vi "lookup_edge.vi"(9 "destination":refnum<class "Node.lvclass">, 10 "source":refnum<class "Node.lvclass">, 11 "digraph in":refnum<class "Graph.lvclass">) -> (1 "edge":refnum<class "Edge.lvclass">, 2 "edge not found?":bool)   [LabVIEW 2020, in "graph.lvlib" / "Graph.lvclass"]
uses:
  Graph.lvclass
  Node/Node.lvclass
  Edge/Edge.lvclass
  Node/Node.lvclass/Node.ctl
  Graph.lvclass/Graph.ctl
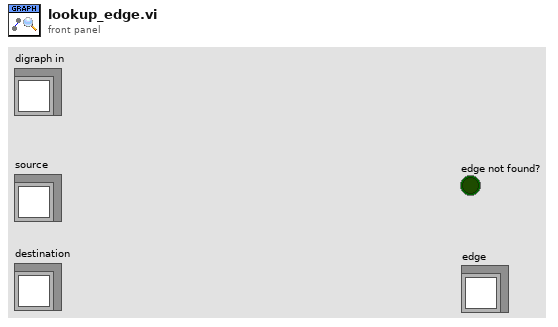
[diagram p1: front panel]
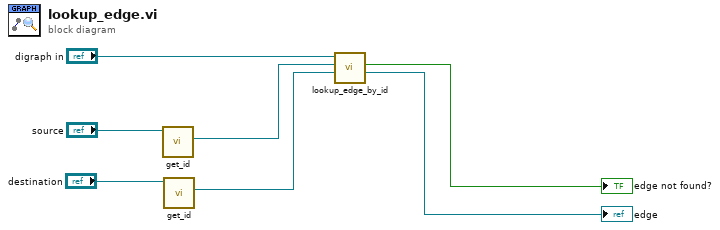
[diagram p0: block diagram]
diagram:
  n1 = call "get_id.vi"("node"="source") -> ("node-id"=w2:refnum<class "ID.lvclass">)  [unwired: 10 in]
  n2 = call "get_id.vi"("node"="destination") -> ("node-id"=w1:refnum<class "ID.lvclass">)  [unwired: 10 in]
  n3 = call "lookup_edge_by_id.vi"("destination_id"=w1, "source_id"=w2, "graph"="digraph in") -> ("edge"=→"edge":refnum<class "Edge.lvclass">, "edge not found?"=→"edge not found?":bool)  [unwired: 7 in]
